vi "Tusk.SetName (Local).vi"(8 "error in (no error)":errorcluster, 10 "Name":string, 11 "Tusk in":refnum<class "Tusk.lvclass">) -> (0 "error out":errorcluster, 3 "Tusk out":refnum<class "Tusk.lvclass">)   [LabVIEW 2018, in "Application.lvlib" / "Tusk.lvclass"]
uses:
  Tusk.lvclass
  Tusk.lvclass/Tusk.ctl
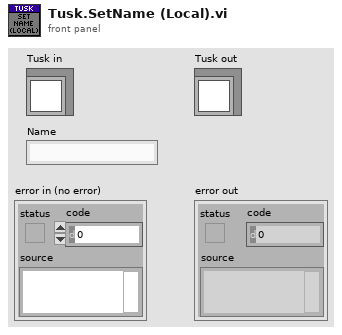
[diagram p1: front panel]
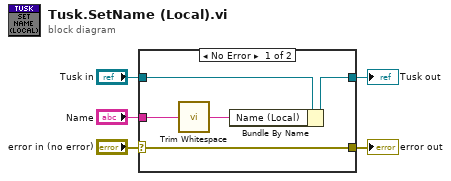
[diagram p0: block diagram]
diagram:
  n1 = case shown="No Error" "error in (no error)" {
    selector: "error in (no error)" -> [w10 w12]
    tunnel: [w10 w12] -> w4
    tunnel: [w6 w11] -> w2
    tunnel: "Tusk in" -> [w8 w11]
    tunnel: "Name" -> [w9 _]
    frame No Error {
      n2 = call <vilib>:"Trim Whitespace.vi"("string"=w9) -> ("trimmed string"=w7:string)  [unwired: 1 in]
      n3 = Bundle By Name(cluster=w8, "Name (Local)"=w7) -> (w6:refnum<class "Tusk.lvclass">)
    }
    frame Error {
    }
  }
  "error out" <- w4
  "Tusk out" <- w2
